vi "Modulation d'amplitude.vi"() -> ()   [LabVIEW 2014]
panel:
  in  "temps":dbl(knob) scale=0.0..1000.0
  out "modulé Graph 3":dynamicdata(graph)
  out "Porteuse Graph 2":dynamicdata(graph)
  out "message Graph":dynamicdata(graph)
  in  "indice de Modulation":dbl(knob) scale=0.0..2.0
  in  "freq porteuse":dbl(knob) scale=0.0..1000.0
  in  "freq message":dbl(knob) scale=0.0..100.0
  in  "stop":bool
  # "y(t)=(1+m.sin(wmt)).Ac.sin(wct)"
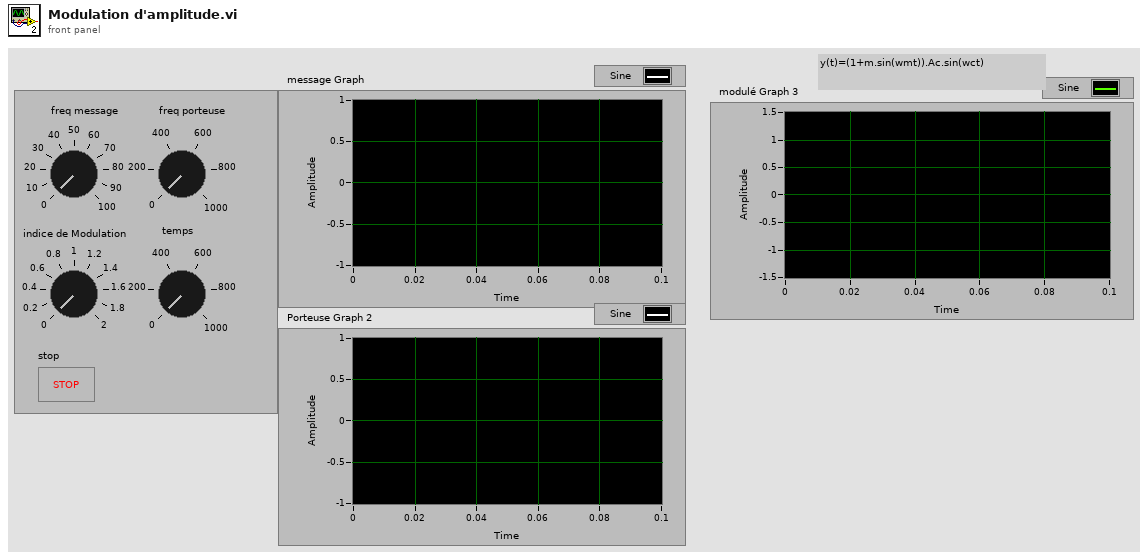
[diagram p1: front panel]
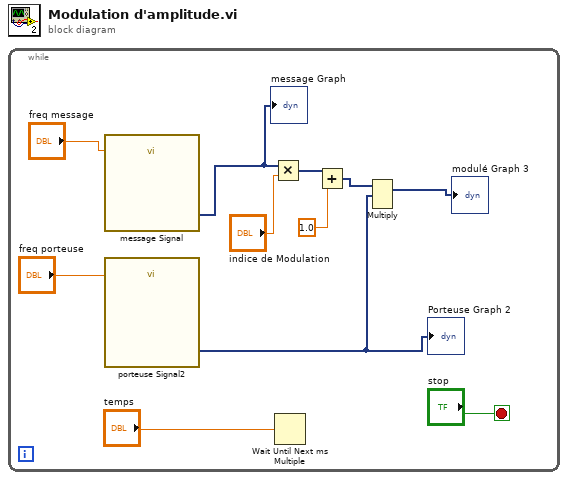
[diagram p0: block diagram]
diagram:
  n1 = while {
    stop <- "stop" stop-if-true
    n2 = call "message Signal"("Frequency"="freq message") -> ("Sine"=w2:dynamicdata)  [unwired: 13 in, 1 out]
    "message Graph" <- w2
    n3 = call "porteuse Signal2"("Frequency"="freq porteuse") -> ("Sine"=w4:dynamicdata)  [unwired: 13 in, 1 out]
    "Porteuse Graph 2" <- w4
    n4 = Multiply(x=w2, y="indice de Modulation") -> (x*y=w7:dynamicdata)
    n5 = Wait Until Next ms Multiple(millisecond multiple="temps") -> ()  [unwired: 1 out]
    n6 = Add(x=w7, y=1.0) -> (x+y=w5:dynamicdata)
    n7 = Multiply(1:w4, 2:w5) -> (0:→"modulé Graph 3":dynamicdata)  [unwired: 1 in, 1 out]
  }
